vi "Display Info.vi"(7 "Layout ref":refnum<vi>, 8 "error in (no error)":errorcluster, 9 "Modify (F) /Add [T]":bool=TRUE, 10 "Names in use":string[](array[string])=["PB"], 11 "Aerotech_Soloist in":refnum<class "Aerotech_Soloist.lvclass">=refnum) -> (0 "error out":errorcluster, 1 "Names in use out":string[](array[string])=["PB"], 2 "Changes Made?":bool=TRUE, 3 "Aerotech_Soloist out":refnum<class "Aerotech_Soloist.lvclass">)   [LabVIEW 2013, in "Aerotech_Soloist.lvclass"]
uses:
  Aerotech_Soloist.lvclass
  ColumnVIs/MenuDisableCol/MenuDisableCol.lvclass
  ColumnVIs/MenuCol/MenuCol.lvclass
  ColumnVIs/Column/Column.lvclass
  ParameterSet.ctl
  TypeDefs/ColumnAppearCluster.ctl
  Aerotech_Soloist.lvclass/Aerotech_Soloist.ctl
panel:
  in  "Change All Appearances":T1={"Column Name"="Command", "Width"=90, "Bkgd"=[16448250, 16770626], "Text"=[0]}
  in  "Feedrate Appearance":T1={"Column Name"="Feedrate", "Width"=30, "Bkgd"=[16448250], "Text"=[0]}
  in  "Pos'n Appearance":T1={"Column Name"="Position", "Width"=30, "Bkgd"=[16448250], "Text"=[0]}
  in  "Parameters Appearance":T1={"Column Name"="Parameters", "Width"=90, "Bkgd"=[16448250, 16770626], "Text"=[0]}
  in  "Command Appearance":T1={"Column Name"="Command", "Width"=90, "Bkgd"=[16448250, 16770626], "Text"=[0]}
  in  "Cancel":bool
  in  "Done":bool
  in  "Device Description":string="Aerotech airstage motion controller"
  in  "Name":string="AeroTech Soloist"
  in  "ParameterList":T2[](array[typedef])=[{"Name"="Default", "SCurve %"=50.0, "Ramp Mode"="RATE", "Ramp Value"=100.0}] {"SCurve %" min=0.0 max=100.0}
  in  "Master Channel":i32=65535
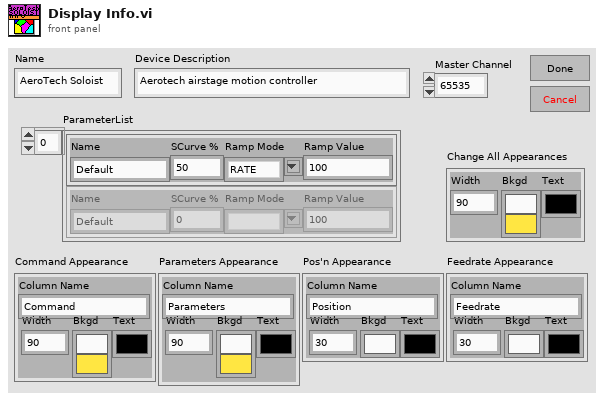
[diagram p1: front panel]
types:
  T1 = typedef "ColumnAppearCluster.ctl" = cluster{"Column Name":string, "Width":u32, "Bkgd":u32[], "Text":u32[]}
  T2 = typedef "Aerotech_Soloist.lvclass/ParameterSet.ctl" = cluster{"Name":string, "SCurve %":dbl, "Ramp Mode":string, "Ramp Value":dbl}
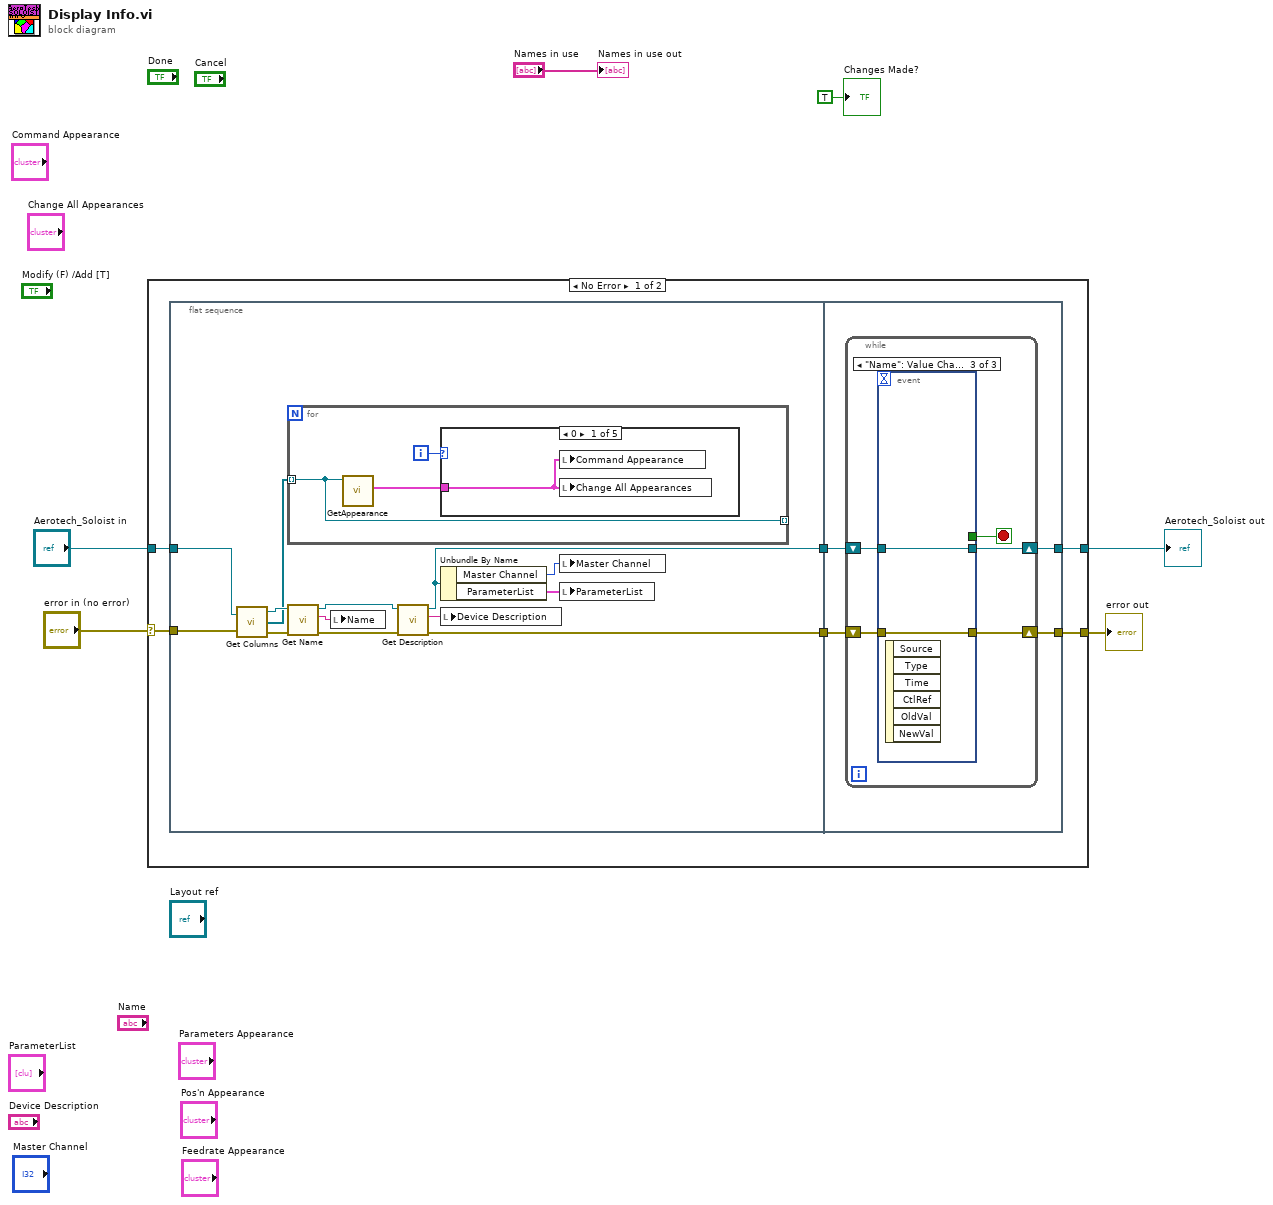
[diagram p0: block diagram]
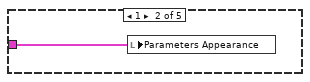
[diagram p2: hidden frame]
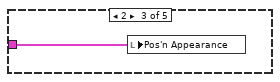
[diagram p3: hidden frame]
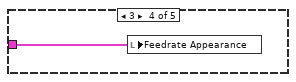
[diagram p4: hidden frame]
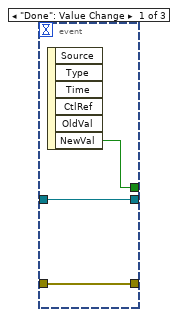
[diagram p6: hidden frame]
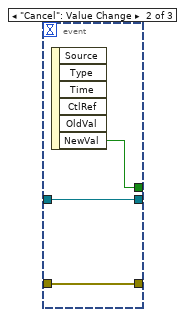
[diagram p7: hidden frame]
diagram:
  n1 = case shown="No Error" "error in (no error)" {
    selector: "error in (no error)" -> [w9 w50]
    tunnel: "Aerotech_Soloist in" -> [w12 w51]
    tunnel: [w11 w51] -> w4
    tunnel: [w10 w50] -> w2
    frame No Error {
      n2 = flat-sequence {
        tunnel: w12 -> [w25]
        tunnel: w9 -> [w13]
        tunnel: [w15] -> w8
        tunnel: [w14] -> w7
        tunnel: [w33] -> w10
        tunnel: [w36] -> w11
        tunnel: w8 -> [w35]
        tunnel: w7 -> [w34]
        frame #0 {
          n3 = call-dynamic "Get Columns.vi"("Device in"=w25, "error in (no error)"=w13) -> ("Device out"=w24:refnum<class "Aerotech_Soloist.lvclass">, "Columns"=w16:refnum<class "Column.lvclass">[], "error out"=w19:errorcluster)
          n4 = for {
            tunnel: [w28] -> _ mode=indexing
            tunnel: w16 -> [w28] mode=indexing
            i -> [w27]
            n5 = call "GetAppearance.vi"("Column in"=w28) -> ("Column Appearance"=w26:T1)  [unwired: 8 in, 2 out]
            n6 = case shown="0" w27 {
              tunnel: w26 -> [w29 w30 w31 w32 _]
              frame 0 {
                n7 = local write "Command Appearance"(w29) -> ()
                n8 = local write "Change All Appearances"(w29) -> ()
              }
              frame 1 {
                n9 = local write "Parameters Appearance"(w30) -> ()
              }
              frame 2 {
                n10 = local write "Pos'n Appearance"(w31) -> ()
              }
              frame 3 {
                n11 = local write "Feedrate Appearance"(w32) -> ()
              }
              frame Default {
              }
            }
          }
          n12 = call-dynamic "Get Name.vi"("error in (no error)"=w19, "Device in"=w24) -> ("error out"=w20:errorcluster, "Name"=w22:string, "Device out"=w23:refnum<class "Aerotech_Soloist.lvclass">)  [unwired: 7 in]
          n13 = local write "Name"(w22) -> ()
          n14 = call-dynamic "Get Description.vi"("error in (no error)"=w20, "Device in"=w23) -> ("error out"=w14:errorcluster, "Device Description"=w21:string, "Device out"=w15:refnum<class "Aerotech_Soloist.lvclass">)  [unwired: 7 in]
          n15 = Unbundle By Name(w15) -> ("Master Channel"=w17:i32, "ParameterList"=w18:T2[])
          n16 = local write "Device Description"(w21) -> ()
          n17 = local write "Master Channel"(w17) -> ()
          n18 = local write "ParameterList"(w18) -> ()
        }
        frame #1 {
          n19 = while {
            shift-right: [w39] -> w36
            shift-left: w35 -> [w40]
            shift-right: [w37] -> w33
            shift-left: w34 -> [w38]
            stop <- w41 stop-if-true
            n20 = event shown="[2] \"Name\": Value Change" {
              selector: _ -> [_ _ _]
              dyn-events: _ -> [_ _ _]
              timeout: _ -> [_ _ _]
              tunnel: [w44 w47 _] -> w41
              tunnel: w40 -> [w43 w46 w49]
              tunnel: [w43 w46 w49] -> w39
              tunnel: w38 -> [w42 w45 w48]
              tunnel: [w42 w45 w48] -> w37
              event "Done": Value Change {
                n21 = event-data() -> ("NewVal"=w44:bool)  [unwired: 1 in, 5 out]
              }
              event "Cancel": Value Change {
                n22 = event-data() -> ("NewVal"=w47:bool)  [unwired: 1 in, 5 out]
              }
              event "Name": Value Change {
                n23 = event-data() -> ()  [unwired: 1 in, 6 out]
              }
            }
          }
        }
      }
    }
    frame Error {
    }
  }
  "error out" <- w2
  "Aerotech_Soloist out" <- w4
  "Changes Made?" <- TRUE ("Changes Made?")
  "Names in use out" <- "Names in use"
